vi "byteArrayToString.vi"(6 "lengthPrepended":bool, 8 "error in (no error)":errorcluster, 9 "startIndex":i32, 10 "ByteArrayIn":u8[](array[numeric])) -> (0 "error out":errorcluster, 1 "endIndex":i32, 2 "ByteArrayOut":u8[](array[numeric]), 3 "String":string)   [LabVIEW 2013, in "BSON.lvlib"]
uses:
  BSON.lvlib
  status.ctl
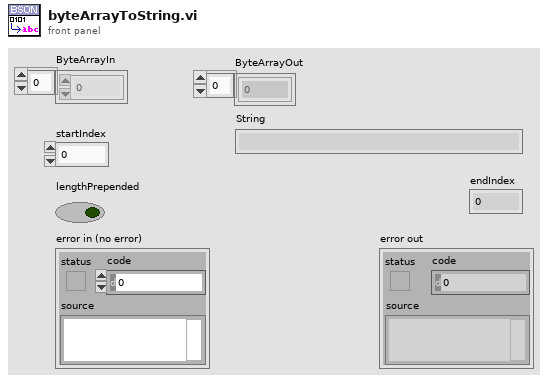
[diagram p1: front panel]
types:
  T1 = typedef "BSON.lvlib/status.ctl" = enum16{"Stream Corrupted or Ended Abruptly", "Incorrect Type In Stream", "ObjectID Invalid", "Method Not Implemented", "Invalid Name", "Invalid URI", "AutoReconnect", "Operation Failed", "Incorrectly Configured", "Cursor Not Found", "Timeout", "Invalid Type", "Empty Name", "Duplicate Name", "MD5Incorrect"}
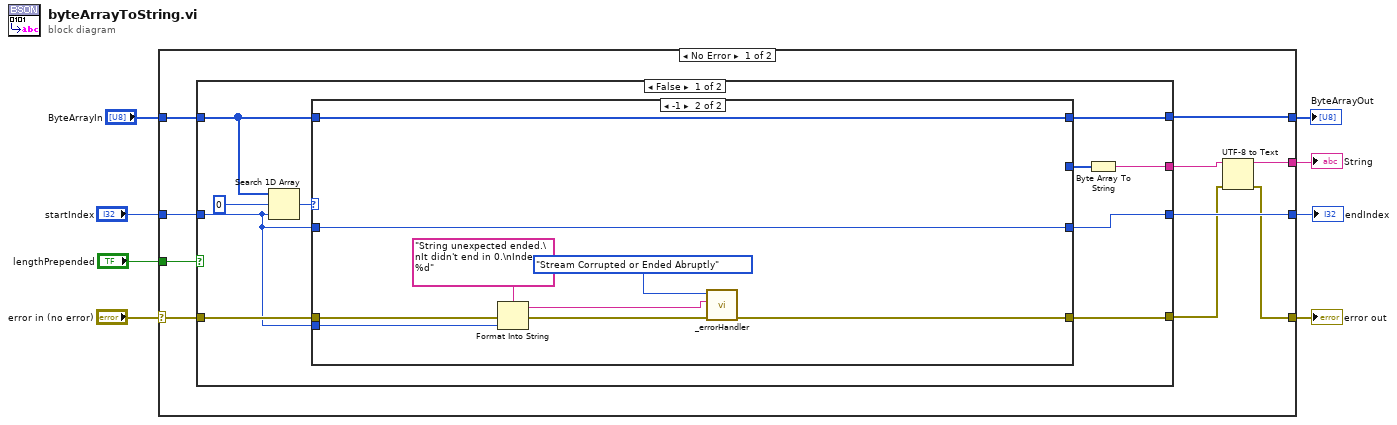
[diagram p0: block diagram]
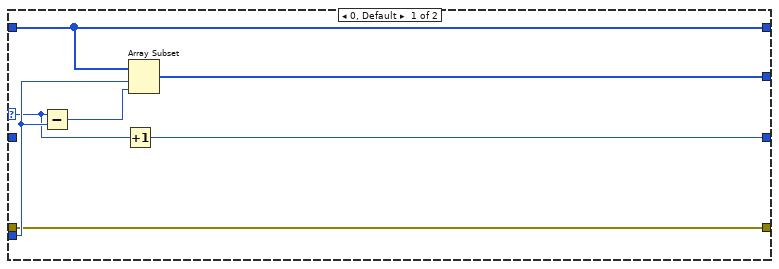
[diagram p2: hidden frame]
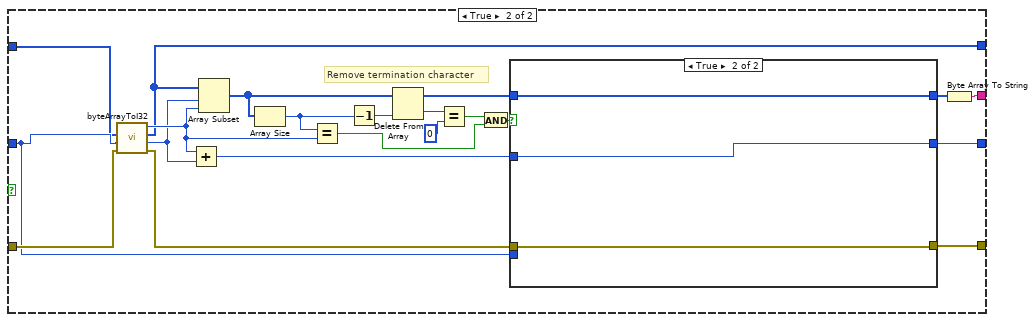
[diagram p3: hidden frame]
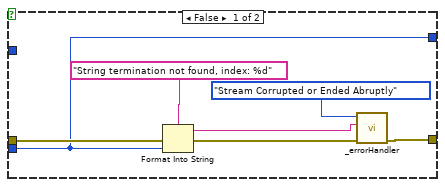
[diagram p4: hidden frame]
diagram:
  n1 = case shown="No Error" "error in (no error)" {
    selector: "error in (no error)" -> [w12 w78]
    tunnel: "ByteArrayIn" -> [w18 w76]
    tunnel: [w14 w78] -> w7
    tunnel: [w17 _] -> w6
    tunnel: "startIndex" -> [w16 w77]
    tunnel: "lengthPrepended" -> [w13 _]
    tunnel: [w15 w77] -> w3
    tunnel: [w9 w76] -> w1
    frame No Error {
      n2 = case shown="False" w13 {
        tunnel: w18 -> [w25 w49]
        tunnel: w16 -> [w23 w50]
        tunnel: [w24 w54] -> w15
        tunnel: w12 -> [w26 w52]
        tunnel: [w22 w53] -> w11
        tunnel: [w19 w46] -> w10
        tunnel: [w21 w45] -> w9
        frame False {
          n3 = Search 1D Array(1D array=w25, element=u8 0, start index (0)=w23) -> (index of element=w27:i32)
          n4 = case shown="-1" w27 {
            selector: w27 -> [w31 _]
            tunnel: w26 -> [w34 w43]
            tunnel: w23 -> [w35 w39]
            tunnel: w25 -> [w29 w36]
            tunnel: [w33 w38] -> w24
            tunnel: [w32 _] -> w20
            tunnel: w23 -> [_ w38]
            tunnel: [w34 w37] -> w22
            tunnel: [w29 w36] -> w21
            frame 0, Default {
              n5 = Subtract(x=w31, y=w35) -> (x-y=w30:i32)
              n6 = Increment(x=w31) -> (x+1=w33:i32)
              n7 = Array Subset(array=w29, index=w35, length=w30) -> (w32:u8[])
            }
            frame -1 {
              n8 = Format Into String(format string="String unexpected ended.\nIt didn't end in 0.\nIndex: %d" ("Additional Text"), error in=w43, w39) -> (resulting string=w40:string, error out=w41:errorcluster)  [unwired: 1 in]
              n9 = call "_errorHandler.vi"("error in (no error)"=w41, "Additional Text"=w40, "Error Type"=status."Stream Corrupted or Ended Abruptly") -> ("error out"=w37:errorcluster)  [unwired: 8 in]
            }
          }
          n10 = Byte Array To String(unsigned byte array=w20) -> (string=w19:string)
        }
        frame True {
          # "Remove termination character"
          n11 = call "byteArrayToI32.vi"("error in (no error)"=w52, "StartIndex"=w50, "ByteArrayIn"=w49) -> ("error out"=w51:errorcluster, "EndIndex"=w48:i32, "ByteArrayOut"=w45:u8[], "I32"=w65:i32)  [unwired: 5 in]
          n12 = Add(x=w65, y=w48) -> (x+y=w56:i32)
          n13 = Array Subset(array=w45, index=w48, length=w65) -> (w59:u8[])
          n14 = Array Size(array=w59) -> (size(s)=w64:i32)
          n15 = Equal?(x=w64, y=w65) -> (x = y?=w58:bool)
          n16 = Decrement(x=w64) -> (x-1=w60:i32)
          n17 = Delete From Array(array=w59, index=w60) -> (deleted portion=w61:u8, array with subset deleted=w55:u8[])  [unwired: 1 in]
          n18 = Equal?(x=w61, y=u8 0) -> (x = y?=w63:bool)
          n19 = And(x=w63, y=w58) -> (x .and. y?=w57:bool)
          n20 = case shown="True" w57 {
            tunnel: w56 -> [_ w74]
            tunnel: w55 -> [_ w75]
            tunnel: [_ w75] -> w47
            tunnel: [w67 w74] -> w54
            tunnel: w51 -> [w68 w73]
            tunnel: w50 -> [w67 _]
            tunnel: [w66 w73] -> w53
            frame False {
              n21 = Format Into String(format string="String termination not found, index: %d" ("Additional Text"), error in=w68, w67) -> (resulting string=w69:string, error out=w70:errorcluster)  [unwired: 1 in]
              n22 = call "_errorHandler.vi"("error in (no error)"=w70, "Additional Text"=w69, "Error Type"=status."Stream Corrupted or Ended Abruptly") -> ("error out"=w66:errorcluster)  [unwired: 8 in]
            }
            frame True {
            }
          }
          n23 = Byte Array To String(unsigned byte array=w47) -> (string=w46:string)
        }
      }
      n24 = UTF-8 to Text(8:w11, 11:w10) -> (0:w14:errorcluster, 3:w17:string)
    }
    frame Error {
    }
  }
  "String" <- w6
  "error out" <- w7
  "endIndex" <- w3
  "ByteArrayOut" <- w1
